vi "Get LB Semaphore.vi"(4 "action (Get)":T1=enum."Get", 5 "error in":errorcluster, 8 "LB reference in":refnum<vi>) -> (0 "error out":errorcluster, 1 "SerSemDict":variant, 2 "semaphore out":T2, 3 "LB reference out":refnum<vi>)   [LabVIEW 2020]
doc: "Developed by Kevin Thompson\nkevin@thompsonengineering.net\n\nCopyright 2013\nThompson Engineering, LLC"
uses:
  TD GetSemaphore Action--enum.ctl
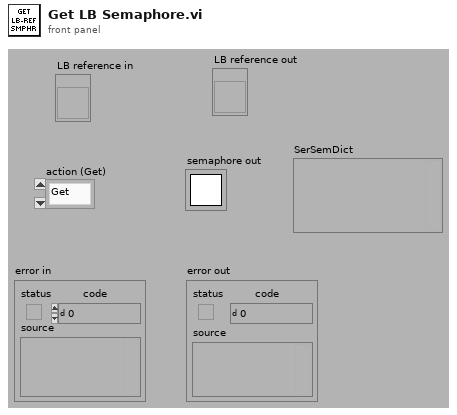
[diagram p1: front panel]
types:
  T1 = typedef "TD GetSemaphore Action--enum.ctl" = enum16{"Init", "Get", "NoOp"}
  T2 = typedef "Semaphore RefNum" = refnum<k1>
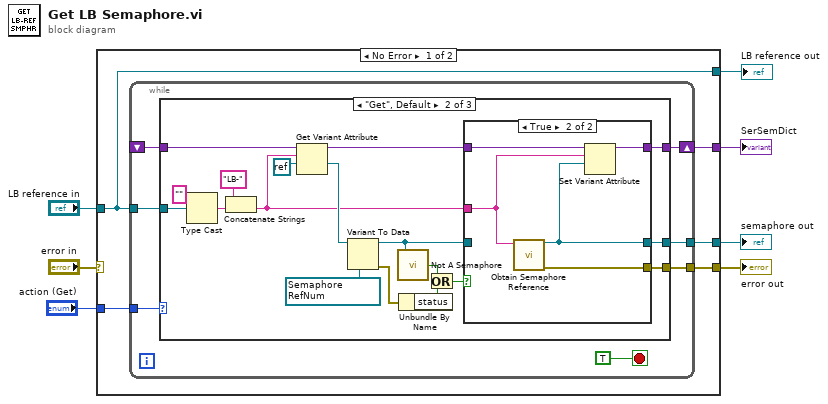
[diagram p0: block diagram]
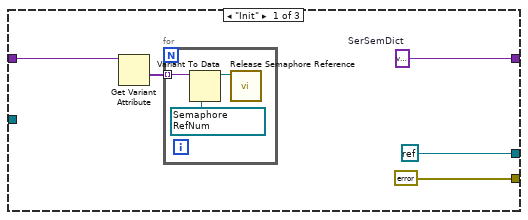
[diagram p2: hidden frame]
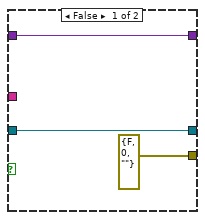
[diagram p3: hidden frame]
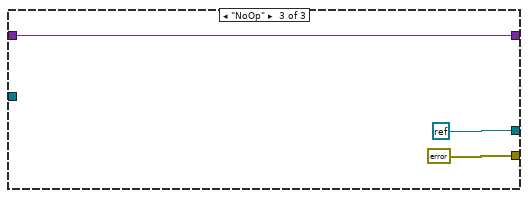
[diagram p4: hidden frame]
diagram:
  n1 = case shown="No Error" "error in" {
    selector: "error in" -> [_ w58]
    tunnel: "LB reference in" -> [w10 w57]
    tunnel: [w9 _] -> w5
    tunnel: [w12 w58] -> w6
    tunnel: "action (Get)" -> [w11 _]
    tunnel: [w10 w57] -> w2
    tunnel: [w8 _] -> w1
    frame No Error {
      n2 = while {
        tunnel: w10 -> [w19]
        tunnel: [w17] -> w12
        shift-right: [w15] -> w8
        shift-left: _ -> [w14]
        tunnel: w11 -> [w16]
        tunnel: [w13] -> w9
        stop <- TRUE stop-if-true
        n3 = case shown="\"Get\", Default" w16 {
          tunnel: [refnum<k0> refnum w45 refnum<k0> refnum] -> w13
          tunnel: w19 -> [_ w41 _]
          tunnel: [errorcluster {"status"=FALSE, "code"=0, "source"=""} ("error out") w44 errorcluster {"status"=FALSE, "code"=0, "source"=""} ("error out")] -> w17
          tunnel: [w24 w43 w56] -> w15
          tunnel: w14 -> [w21 w32 w56]
          frame "Init" {
            w24 = variant  # SerSemDict
            n4 = Get Variant Attribute(Variant=w21) -> (values=w20:variant[])  [unwired: 3 in, 3 out]
            n5 = for {
              tunnel: w20 -> [w27] mode=indexing
              w25 = T2 refnum items=["semaphore"] ("semaphore")
              n6 = Variant To Data(type=w25, Variant=w27) -> (data=w26:T2)  [unwired: 1 in, 1 out]
              n7 = call <vilib>:"Release Semaphore Reference.vi"("semaphore"=w26) -> ()  [unwired: 9 in, 2 out]
            }
          }
          frame "Get", Default {
            w39 = T2 refnum items=["semaphore"] ("semaphore")
            n8 = Type Cast(type="", x=w41) -> (*(type *) &x=w30:string)
            n9 = Concatenate Strings("LB-" ("string"), w30) -> (w28:string)
            n10 = Get Variant Attribute(Variant=w32, name=w28, default value (empty Variant)=refnum<k0> refnum) -> (duplicate Variant=w31:variant, value=w38:refnum<k0>)  [unwired: 1 in, 2 out]
            n11 = Variant To Data(type=w39, Variant=w38) -> (data=w37:T2, error out=w36:errorcluster)  [unwired: 1 in]
            n12 = call <vilib>:"Not A Semaphore.vi"("semaphore"=w37) -> ("not a semaphore"=w33:bool)
            n13 = Unbundle By Name(w36) -> ("status"=w35:bool)
            n14 = Or(x=w33, y=w35) -> (x .or. y?=w34:bool)
            n15 = case shown="True" w34 {
              tunnel: [w47 w50] -> w45
              tunnel: [errorcluster {"status"=FALSE, "code"=0, "source"=""} ("error out") w53] -> w44
              tunnel: w31 -> [w46 w52]
              tunnel: [w46 w51] -> w43
              tunnel: w28 -> [_ w49]
              tunnel: w37 -> [w47 _]
              frame False {
              }
              frame True {
                n16 = call <vilib>:"Obtain Semaphore Reference.vi"("name (unnamed)"=w49) -> ("error out"=w53:errorcluster, "semaphore"=w50:T2)  [unwired: 4 in, 1 out]
                n17 = Set Variant Attribute(Variant=w52, name=w49, value=w50) -> (Variant out=w51:variant)  [unwired: 1 in, 2 out]
              }
            }
          }
          frame "NoOp" {
          }
        }
      }
    }
    frame Error {
    }
  }
  "error out" <- w6
  "semaphore out" <- w5
  "LB reference out" <- w2
  "SerSemDict" <- w1
